vi "Build Port ID Message.vi"(9 "Assert ID String":string, 11 "New Port Number":u16) -> (2 "Assert Port ID Message":string)   [LabVIEW 2016, in "Assert API Components.lvlib" / "Assert Service.lvlib" / "UDP Listener.lvclass"]
doc: "Builds up a unique ID message out of the assert ID string and the newly requested port number"
uses:
  UDP Listener.lvclass
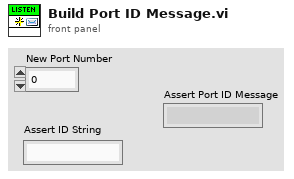
[diagram p1: front panel]
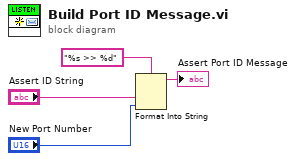
[diagram p0: block diagram]
diagram:
  n1 = Format Into String(format string="%s >> %d", "Assert ID String", "New Port Number") -> (resulting string=→"Assert Port ID Message":string)  [unwired: 2 in, 1 out]
